vi "水质测量数据table定义.vi"(5 "数据标记表":string(combo)="N", 7 "table 输入":string, 9 "SN":string, 10 "测量模式":T1(ring)=enum."水样测试", 11 "data":T3 {"单位" items=["ug/L", "mg/L", "ppm", "mg/m3", "cm", "ppb", "ug/m3", "%", "nmol/mol", "umol/mol", "MPN/L", "MPN/100ml", "ng/m3", "NTU", "无量纲", "ms/cm", "us/cm"]}) -> (1 "table 输出":string, 2 "columns":string[](array[string]), 3 "data输出":T2)   [LabVIEW 2016, in "database.lvlib"]
uses:
  database.lvlib
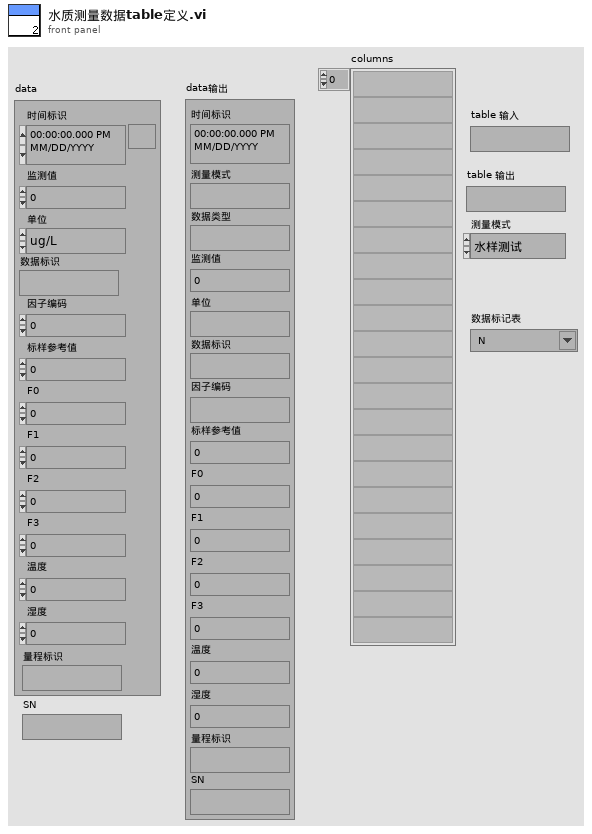
[diagram p1: front panel]
types:
  T1 = enum16{"维护数据", "水样测试", "标样核查", "零点核查", "跨度核查", "空白测试", "平行样测试", "加标回收", "空白校准", "标样校准", "初始化（清洗）"}
  T2 = cluster{"时间标识":timestamp, "测量模式":string, "数据类型":string, "监测值":sgl, "单位":string, "数据标识":string, "因子编码":string, "标样参考值":sgl, "F0":sgl, "F1":sgl, "F2":sgl, "F3":sgl, "温度":sgl, "湿度":sgl, "量程标识":string, "SN":string}
  T3 = cluster{"时间标识":timestamp, "监测值":sgl, "单位":u16, "数据标识":string, "因子编码":u32, "标样参考值":sgl, "F0":sgl, "F1":sgl, "F2":sgl, "F3":sgl, "温度":sgl, "湿度":sgl, "量程标识":string}
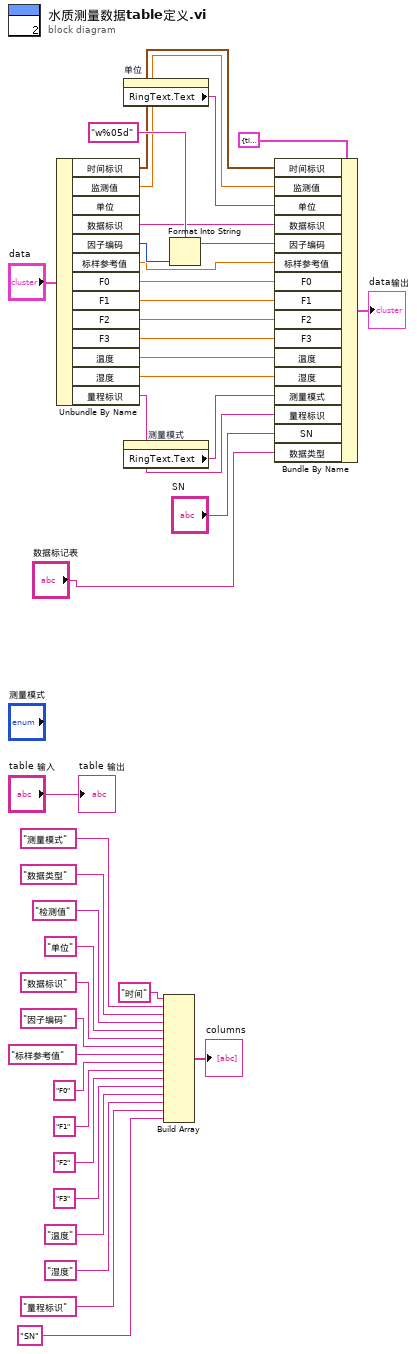
[diagram p0: block diagram]
diagram:
  n1 = Unbundle By Name("data") -> ("时间标识"=w23:timestamp, "监测值"=w22:sgl, "数据标识"=w21:string, "因子编码"=w27:u32, "标样参考值"=w12:sgl, "F0"=w13:sgl, "F1"=w20:sgl, "F2"=w19:sgl, "F3"=w18:sgl, "温度"=w17:sgl, "湿度"=w16:sgl, "量程标识"=w7:string)  [unwired: 1 out]
  n2 = property on="单位" class="Ring (严格)"() -> ("RingText.Text"=w15:string)  [unwired: 2 in, 2 out]
  n3 = property on="测量模式" class="Enum (严格)"() -> ("RingText.Text"=w9:string)  [unwired: 2 in, 2 out]
  n4 = Build Array("时间", "测量模式", "数据类型", "检测值", "单位", "数据标识", "因子编码", "标样参考值", "F0", "F1", "F2", "F3", "温度", "湿度", "量程标识", "SN") -> (→"columns":string[])
  n5 = Format Into String(format string="w%05d" ("格式字符串"), w27) -> (resulting string=w24:string)  [unwired: 2 in, 1 out]
  n6 = Bundle By Name(cluster=T2 {"时间标识"=timestamp(0 s since 1904-01-01), "测量模式"="", "数据类型"="", "监测值"=0.0, "单位"="", "数据标识"="", "因子编码"="", "标样参考值"=0.0, "F0"=0.0, "F1"=0.0, "F2"=0.0, "F3"=0.0, "温度"=0.0, "湿度"=0.0, "量程标识"="", "SN"=""} ("data输出"), "时间标识"=w23, "监测值"=w22, "单位"=w15, "数据标识"=w21, "因子编码"=w24, "标样参考值"=w12, "F0"=w13, "F1"=w20, "F2"=w19, "F3"=w18, "温度"=w17, "湿度"=w16, "测量模式"=w9, "量程标识"=w7, "SN"="SN", "数据类型"="数据标记表") -> (→"data输出":T2)
  "table 输出" <- "table 输入"
